vi "INIpath.vi"() -> (2 "INI File path":path, 3 "ServerLog path":path)   [LabVIEW 2017, in "Server.lvlib"]
doc: "This VI outputs the Path to the INI-File."
uses:
  Server.lvlib
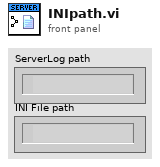
[diagram p1: front panel]
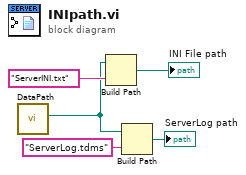
[diagram p0: block diagram]
diagram:
  n1 = call "DataPath.vi"() -> ("DataDirectory"=w3:path)  [unwired: 11 in]
  n2 = Build Path(base path=w3, name or relative path="ServerINI.txt") -> (appended path=→"INI File path":path)
  n3 = Build Path(base path=w3, name or relative path="ServerLog.tdms") -> (appended path=→"ServerLog path":path)
